vi "GripperSettings.vi"() -> (0 "RC":T1={"SP Left"=172.0, "SP Right"=882.0}, 1 "Cycle":T1={"SP Left"=916.0, "SP Right"=137.0}, 2 "Open":T1={"SP Left"=547.0, "SP Right"=507.0}, 3 "Close":T1={"SP Left"=677.0, "SP Right"=377.0})   [LabVIEW 2014, in "Elevator System.lvlib"]
uses:
  Elevator System.lvlib
  Typedef/GripperNotifierType.ctl
panel:
  in  "Cycle":T1={"SP Left"=239.0, "SP Right"=-240.0}
  in  "RC":dbl=505.0
  in  "Open":dbl=130.0
  in  "Close":T1={"SP Left"=677.0, "SP Right"=377.0}
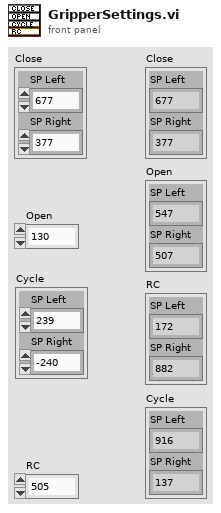
[diagram p1: front panel]
types:
  T1 = typedef "Elevator System.lvlib/GripperNotifierType.ctl" = cluster{"SP Left":dbl, "SP Right":dbl}
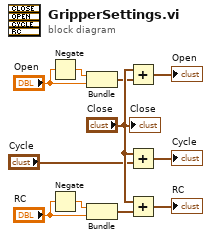
[diagram p0: block diagram]
diagram:
  n1 = Negate(x="Open") -> (-x=w7:dbl)
  n2 = Negate(x="RC") -> (-x=w4:dbl)
  n3 = Bundle(w7, "Open"="Open") -> (w5:cluster{dbl, "Open":dbl})  [unwired: 1 in]
  n4 = Bundle(w4, "RC"="RC") -> (w2:cluster{dbl, "RC":dbl})  [unwired: 1 in]
  n5 = Add(x="Close", y=w5) -> (x+y=→"Open":T1)
  n6 = Add(x="Close", y="Cycle") -> (x+y=→"Cycle":T1)
  n7 = Add(x="Close", y=w2) -> (x+y=→"RC":T1)
  "Close" <- "Close"
